vi "Main.vi"() -> ()   [LabVIEW 2012]
uses:
  Consumer Message.ctl
panel:
  out "State to Execute":string
  out "High Priority?":bool
  out "Backlog":u8(slide) scale=0.0..100.0
  out "Processed Value":i32
  in  "High Priority Message":bool
  in  "Normal Priority Message":bool
  in  "Stop":bool
  # "Number of enqueued\nmessages waiting to\nbe processed"
  # "Current data being\nprocessed in consumer loop"
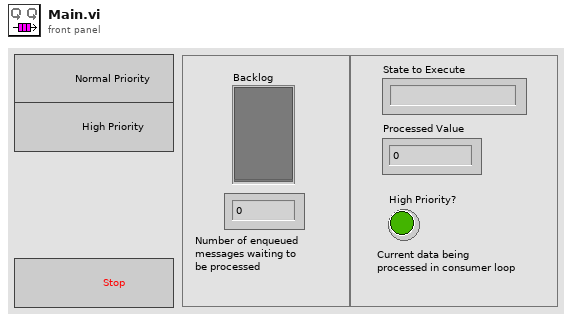
[diagram p1: front panel]
types:
  T1 = typedef "Consumer Message.ctl" = cluster{"Consumer State":string, "Boolean Data":bool, "Numeric Data":i32}
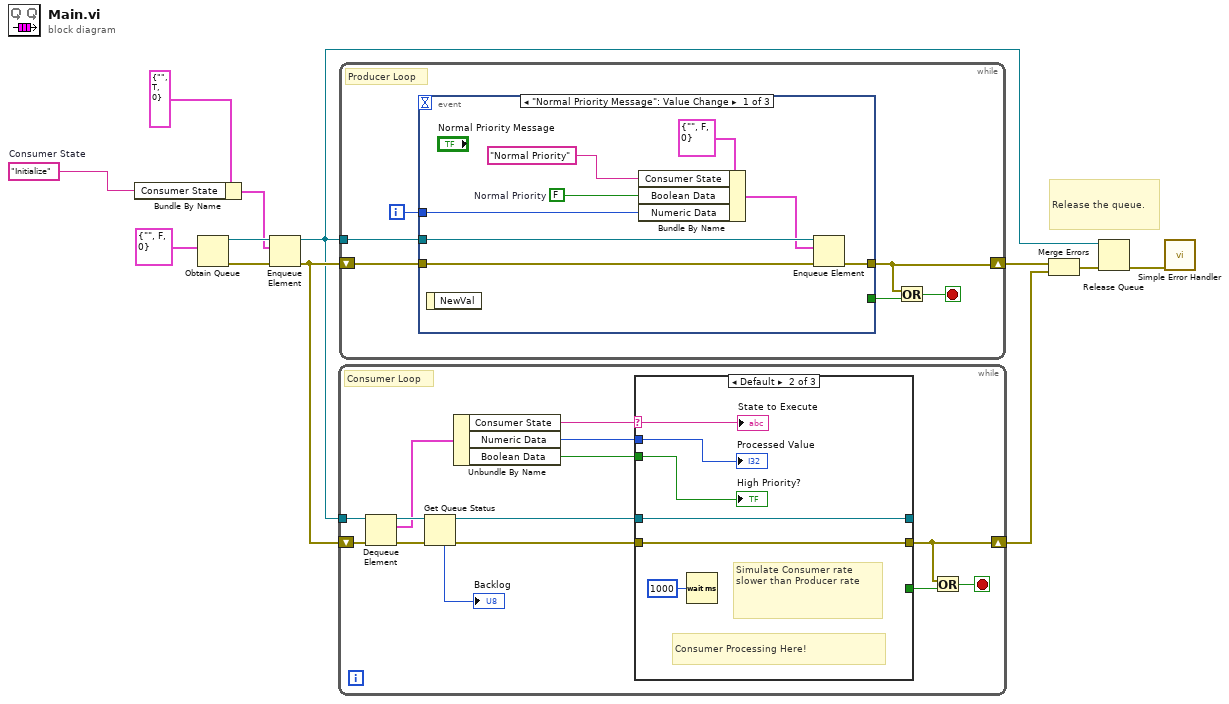
[diagram p0: block diagram]
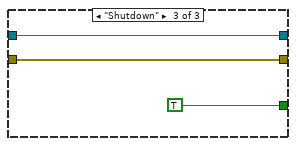
[diagram p3: hidden frame]
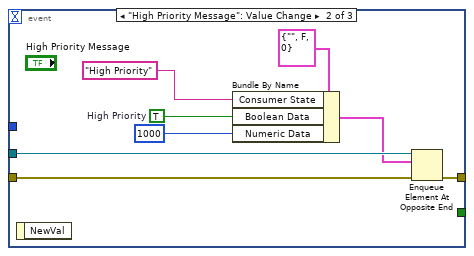
[diagram p4: hidden frame]
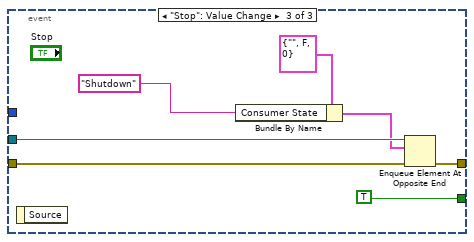
[diagram p5: hidden frame]
diagram:
  w1 = "Initialize"  # Consumer State
  # "Release the queue."
  n1 = Bundle By Name(cluster=T1 {"Consumer State"="", "Boolean Data"=TRUE, "Numeric Data"=0} ("Consumer Message"), "Consumer State"=w1) -> (w2:T1)
  n2 = Obtain Queue(element data type=T1 {"Consumer State"="", "Boolean Data"=FALSE, "Numeric Data"=0}) -> (queue out=w6:refnum<queue>, error out=w12:errorcluster)  [unwired: 4 in, 1 out]
  n3 = Enqueue Element(queue=w6, element=w2, error in (no error)=w12) -> (queue out=w5:refnum<queue>, error out=w7:errorcluster)  [unwired: 1 in, 1 out]
  n4 = while {
    tunnel: w5 -> [w24]
    shift-right: [w13] -> w11
    shift-left: w7 -> [w23]
    stop <- w14 stop-if-true
    # "Consumer Loop"
    n5 = Dequeue Element(queue=w24, error in (no error)=w23) -> (queue out=w25:refnum<queue>, element=w22:T1, error out=w26:errorcluster)  [unwired: 1 in, 1 out]
    n6 = Get Queue Status(queue=w25, error in (no error)=w26) -> (queue out=w16:refnum<queue>, error out=w20:errorcluster, # elements in queue=→"Backlog":i32)  [unwired: 1 in, 5 out]
    n7 = Unbundle By Name(w22) -> ("Consumer State"=w21:string, "Numeric Data"=w19:i32, "Boolean Data"=w17:bool)
    n8 = case shown="Default" w21 {
      selector: w21 -> [_ w31 _]
      tunnel: [_ _ TRUE] -> w15
      tunnel: w20 -> [w27 w29 w35]
      tunnel: [w27 w29 w35] -> w13
      tunnel: w19 -> [_ w34 _]
      tunnel: w17 -> [_ w33 _]
      tunnel: w16 -> [w28 w32 w36]
      tunnel: [w28 w32 w36] -> _
      frame "Initialize" {
      }
      frame Default {
        # "Simulate Consumer rate slower than Producer rate"
        # "Consumer Processing Here!"
        n9 = Wait (ms)(milliseconds to wait=u32 1000) -> ()  [unwired: 1 out]
        "Processed Value" <- w34
        "High Priority?" <- w33
        "State to Execute" <- w31
      }
      frame "Shutdown" {
      }
    }
    n10 = Or(x=w13, y=w15) -> (x .or. y?=w14:bool)
  }
  n11 = while {
    shift-right: [w38] -> w10
    shift-left: w7 -> [w42]
    tunnel: w5 -> [w43]
    i -> [w41]
    stop <- w39 stop-if-true
    # "Producer Loop"
    n12 = event shown="[0] \"Normal Priority Message\": Value Change" {
      selector: _ -> [_ _ _]
      dyn-events: _ -> [_ _ _]
      timeout: _ -> [_ _ _]
      tunnel: w43 -> [w51 w58 w66]
      tunnel: w42 -> [w49 w57 w64]
      tunnel: [w50 w59 w63] -> w38
      tunnel: [_ _ TRUE] -> w40
      tunnel: w41 -> [w48 _ _]
      event "Normal Priority Message": Value Change {
        w45 = FALSE  # Normal Priority
        n13 = event-data() -> ()  [unwired: 1 in, 1 out]
        n14 = Bundle By Name(cluster=T1 {"Consumer State"="", "Boolean Data"=FALSE, "Numeric Data"=0}, "Consumer State"="Normal Priority" ("String Data"), "Boolean Data"=w45, "Numeric Data"=w48) -> (w47:T1)
        n15 = Enqueue Element(queue=w51, element=w47, error in (no error)=w49) -> (error out=w50:errorcluster)  [unwired: 1 in, 2 out]
      }
      event "High Priority Message": Value Change {
        w53 = TRUE  # High Priority
        n16 = event-data() -> ()  [unwired: 1 in, 1 out]
        n17 = Bundle By Name(cluster=T1 {"Consumer State"="", "Boolean Data"=FALSE, "Numeric Data"=0}, "Consumer State"="High Priority" ("String Data"), "Boolean Data"=w53, "Numeric Data"=1000) -> (w55:T1)
        n18 = Enqueue Element At Opposite End(queue=w58, element=w55, error in (no error)=w57) -> (error out=w59:errorcluster)  [unwired: 1 in, 2 out]
      }
      event "Stop": Value Change {
        n19 = event-data() -> ()  [unwired: 1 in, 1 out]
        n20 = Bundle By Name(cluster=T1 {"Consumer State"="", "Boolean Data"=FALSE, "Numeric Data"=0}, "Consumer State"="Shutdown") -> (w60:T1)
        n21 = Enqueue Element At Opposite End(queue=w66, element=w60, error in (no error)=w64) -> (error out=w63:errorcluster)  [unwired: 1 in, 2 out]
      }
    }
    n22 = Or(x=w38, y=w40) -> (x .or. y?=w39:bool)
  }
  n23 = Merge Errors(w10, w11) -> (w9:errorcluster)
  n24 = Release Queue(queue=w5, error in (no error)=w9) -> (error out=w4:errorcluster)  [unwired: 1 in, 2 out]
  n25 = call <vilib>:"Simple Error Handler.vi"("error in (no error)"=w4) -> ()  [unwired: 4 in, 5 out]
